vi "Idle_Reading_Calibration (SubVI).vi"(10 "Dynamic Data":dynamicdata(waveform), 11 "Dynamic Data 2":dynamicdata(waveform)) -> (2 "Cluster":T2, 3 "Cluster 2":T1)   [LabVIEW 2018]
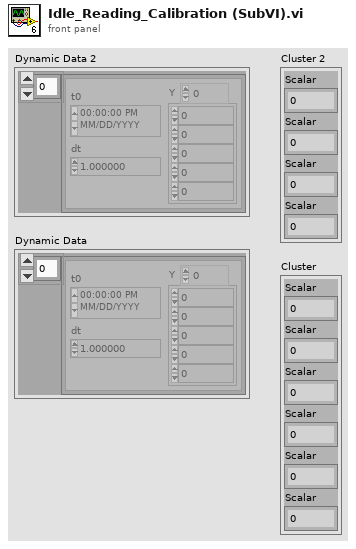
[diagram p1: front panel]
types:
  T1 = cluster{"Scalar":dbl, "Scalar":dbl, "Scalar":dbl, "Scalar":dbl}
  T2 = cluster{"Scalar":dbl, "Scalar":dbl, "Scalar":dbl, "Scalar":dbl, "Scalar":dbl, "Scalar":dbl}
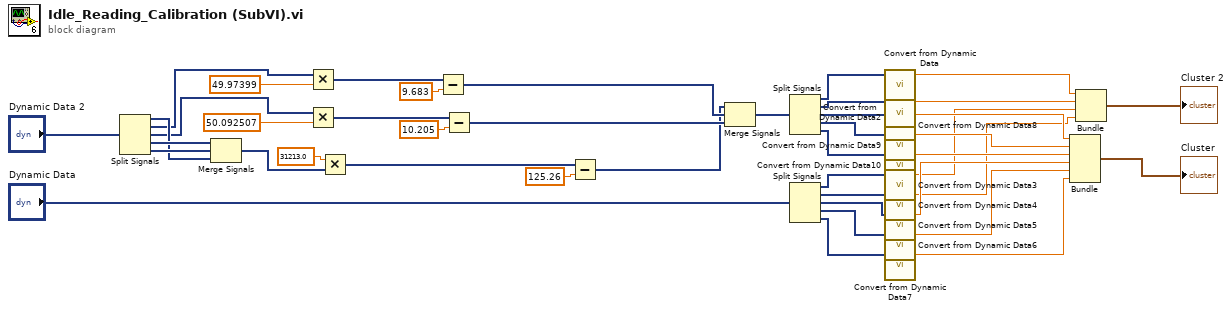
[diagram p0: block diagram]
diagram:
  n1 = Split Signals("Dynamic Data 2") -> (w38:dynamicdata, w33:dynamicdata, w34:dynamicdata, w39:dynamicdata, w40:dynamicdata)  [unwired: 5 in]
  n2 = Merge Signals(w39, w40, w38) -> (w26:dynamicdata)
  n3 = Multiply(x=w33, y=49.97399) -> (x*y=w30:dynamicdata)
  n4 = Multiply(x=w34, y=50.092507) -> (x*y=w27:dynamicdata)
  n5 = Multiply(x=31213.0, y=w26) -> (x*y=w25:dynamicdata)
  n6 = Subtract(x=w30, y=9.683) -> (x-y=w36:dynamicdata)
  n7 = Subtract(x=w27, y=10.205) -> (x-y=w37:dynamicdata)
  n8 = Subtract(x=w25, y=125.26) -> (x-y=w35:dynamicdata)
  n9 = Merge Signals(w35, w36, w37) -> (w41:dynamicdata)
  n10 = Split Signals(w41) -> (w15:dynamicdata, w16:dynamicdata, w17:dynamicdata, w18:dynamicdata, w19:dynamicdata)  [unwired: 5 in]
  n11 = Split Signals("Dynamic Data") -> (w4:dynamicdata, w2:dynamicdata, w7:dynamicdata, w8:dynamicdata, w9:dynamicdata)  [unwired: 5 in]
  n12 = call "Convert from Dynamic Data"("Dynamic Data Type"=w15) -> ("Scalar"=w5:dbl)  [unwired: 3 in]
  n13 = call "Convert from Dynamic Data2"("Dynamic Data Type"=w16) -> ("Scalar"=w6:dbl)  [unwired: 3 in]
  n14 = call "Convert from Dynamic Data8"("Dynamic Data Type"=w17) -> ("Scalar"=w12:dbl)  [unwired: 3 in]
  n15 = call "Convert from Dynamic Data9"("Dynamic Data Type"=w18) -> ("Scalar"=w11:dbl)  [unwired: 3 in]
  n16 = call "Convert from Dynamic Data10"("Dynamic Data Type"=w19) -> ("Scalar"=w10:dbl)  [unwired: 3 in]
  n17 = call "Convert from Dynamic Data3"("Dynamic Data Type"=w4) -> ("Scalar"=w3:dbl)  [unwired: 3 in]
  n18 = call "Convert from Dynamic Data4"("Dynamic Data Type"=w2) -> ("Scalar"=w1:dbl)  [unwired: 3 in]
  n19 = call "Convert from Dynamic Data5"("Dynamic Data Type"=w7) -> ("Scalar"=w13:dbl)  [unwired: 3 in]
  n20 = call "Convert from Dynamic Data6"("Dynamic Data Type"=w8) -> ("Scalar"=w14:dbl)  [unwired: 3 in]
  n21 = call "Convert from Dynamic Data7"("Dynamic Data Type"=w9) -> ("Scalar"=w22:dbl)  [unwired: 3 in]
  n22 = Bundle("Scalar"=w12, "Scalar"=w11, "Scalar"=w10, "Scalar"=w13, "Scalar"=w14, "Scalar"=w22) -> (→"Cluster":T2)  [unwired: 1 in]
  n23 = Bundle("Scalar"=w5, "Scalar"=w6, "Scalar"=w3, "Scalar"=w1) -> (→"Cluster 2":T1)  [unwired: 1 in]
